vi "Write COM.vi"(8 "error in (no error)":errorcluster, 10 "COM":refnum<visa-resource-name>, 11 "OHAUS_Navigator_232 in":refnum<class "OHAUS_Navigator_232.lvclass">) -> (0 "error out":errorcluster, 3 "OHAUS_Navigator_232 out":refnum<class "OHAUS_Navigator_232.lvclass">)   [LabVIEW 2019, in "OHAUS_Navigator_232.lvclass"]
uses:
  OHAUS_Navigator_232.lvclass
  OHAUS_Navigator_232.lvclass/OHAUS_Navigator_232.ctl
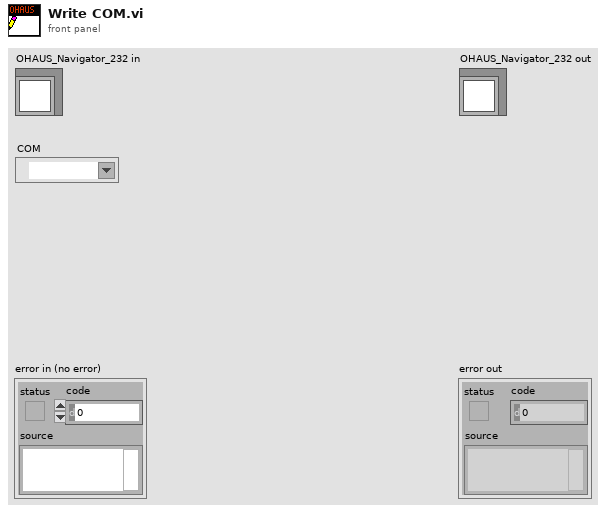
[diagram p1: front panel]
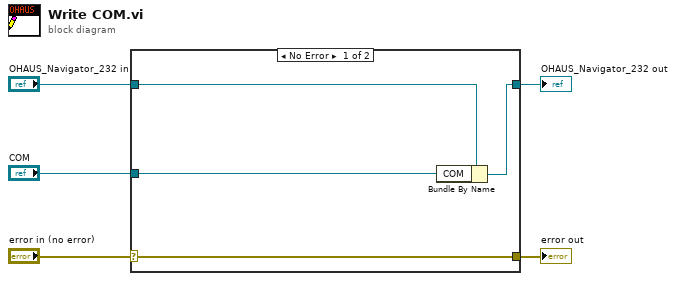
[diagram p0: block diagram]
diagram:
  n1 = case shown="No Error" "error in (no error)" {
    selector: "error in (no error)" -> [w9 w10]
    tunnel: [w9 w10] -> w4
    tunnel: [w7 w11] -> w2
    tunnel: "OHAUS_Navigator_232 in" -> [w8 w11]
    tunnel: "COM" -> [w6 _]
    frame No Error {
      n2 = Bundle By Name(cluster=w8, "COM"=w6) -> (w7:refnum<class "OHAUS_Navigator_232.lvclass">)
    }
    frame Error {
    }
  }
  "error out" <- w4
  "OHAUS_Navigator_232 out" <- w2
